vi "ConversionFORCE.vi"(0 "number":dbl, 2 "number 2":dbl, 3 "number 3":dbl, 5 "number 4":dbl) -> (11 "Torque":dbl, 13 "Vout(Torque)":dbl, 14 "Vout(M)":dbl, 15 "Force(M)":dbl, 16 "Vout(RO)":dbl, 17 "Force(RO)":dbl, 18 "Vout(BO)":dbl, 19 "Force(BO)":dbl)   [LabVIEW 2020]
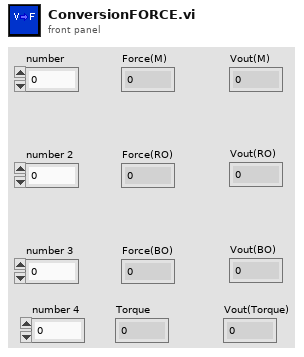
[diagram p1: front panel]
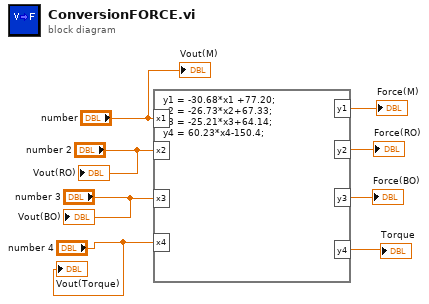
[diagram p0: block diagram]
diagram:
  n1 = formula code="y1 = -30.68*x1 +77.20;\ny2 = -26.73*x2+67.33;\ny3 = -25.21*x3+64.14;\ny4 = 60.23*x4-150.4;"("x1"="number", "x2"="number 2", "x3"="number 3", "x4"="number 4") -> ("y1"=→"Force(M)":dbl, "y2"=→"Force(RO)":dbl, "y3"=→"Force(BO)":dbl, "y4"=→"Torque":dbl)
  "Vout(M)" <- "number"
  "Vout(RO)" <- "number 2"
  "Vout(BO)" <- "number 3"
  "Vout(Torque)" <- "number 4"
